vi "rotmatrix.vi"(8 "alpha":dbl, 10 "phi":dbl, 11 "theta":dbl) -> (1 "matr":dbl[][](array[numeric]))   [LabVIEW 2018]
uses:
  <vilib>/imath/engines/lvmath2/RunTimeEngine/Managers/WorkSpace/UID Generator.vi
  <vilib>/imath/engines/lvmath2/RunTimeEngine/RunTimeType/NIMS_RunTimeType_From StrictType (excl LVString).vi
  <instcachedir>/0/NIMS_RunTimeType_From StrictType (excl LVString)_BB99E21530212246AE80DD055A09BF99.lvgen/NIMS_RunTimeType_From StrictType (excl LVString)_BB99E21530212246AE80DD055A09BF99_000.vi
  <vilib>/imath/engines/lvmath2/RunTimeEngine/LocalVariableDefStatement/MC_LocalVariableDefStatement_Display.vi
  <vilib>/imath/engines/lvmath2/RunTimeEngine/Managers/SymbolTable/Clear UID.vi
  <vilib>/imath/engines/lvmath2/RunTimeEngine/NodeEndStatement/NIMS_NodeEndStatement_Output.vi
  <instcachedir>/0/NIMS_NodeEndStatement_Output_53EC0D466D134D7ABD903AC30B43404B.lvgen/NIMS_NodeEndStatement_Output_53EC0D466D134D7ABD903AC30B43404B_004.vi
  <vilib>/imath/engines/lvmath2/RunTimeEngine/ErrorHandling/NIMS_Finalize Error.vi
  <vilib>/imath/engines/lvmath2/RunTimeEngine/Managers/SymbolTable/NIMS_WorkSpace.lvlib
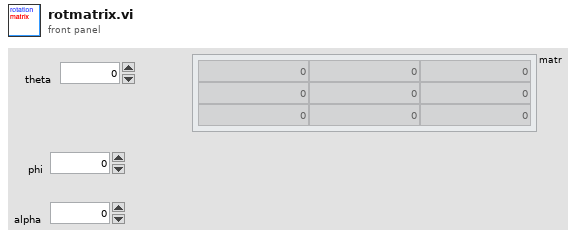
[diagram p1: front panel]
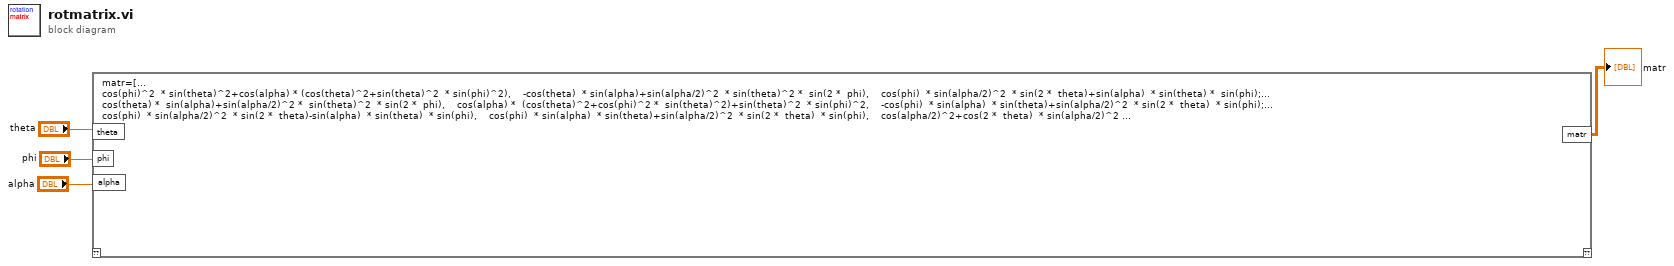
[diagram p0: block diagram]
diagram:
  n1 = mathscript code="matr=[...\ncos(phi)^2  * sin(theta)^2+cos(alpha) * (cos(theta)^2+sin(theta)^2  * sin(phi)^2),\t\t\t\t-cos(theta)  * sin(alpha)+sin(alpha/2)^2  * sin(theta)^2 *  sin(2 *  phi),\t\t\t\tcos(phi)  * sin(alpha/2)^2  * sin(2 *  theta)+sin(alpha)  * sin(theta) *  sin(phi);...\ncos(theta) *  sin(alpha)+sin(alpha/2)^2 *  sin(theta)^2  * sin(2 *  phi),\t\t\t\tcos(alpha) *  (cos(theta)^2+cos(phi)^2 *  sin(theta)^2)+sin(theta)^2  * sin(phi)^2,\t\t\t\t-cos(phi)  * sin(alpha)  * sin(theta)+sin(alpha/2)^2  * sin(2 *  theta)  * sin(phi);...\ncos(phi)  * sin(alpha/2)^2  * sin(2 *  theta)-sin(alpha)  * sin(theta)  * sin(phi),\t\t\t\tcos(phi)  * sin(alpha)  * sin(theta)+sin(alpha/2)^2  * sin(2 *  theta)  * sin(phi),\t\t\t\tcos(alpha/2)^2+cos(2 *  theta)  * sin(alpha/2)^2 ... \n]"("theta"="theta", "phi"="phi", "alpha"="alpha") -> ("matr"=→"matr":dbl[][])  [unwired: 1 in, 1 out]
